vi "Check if configuration files exist.vi"(8 "error in (no error)":errorcluster, 11 "TomoConversionBase in":refnum<class "TomoConversion.lvclass">) -> (0 "error out":errorcluster, 2 "configuration file exists?":bool, 3 "TomoConversionBase out":refnum<class "TomoConversion.lvclass">)   [LabVIEW 2012, in "TomoConversion.lvclass"]
doc: "Checks whether all required configuration files for the component exist."
uses:
  TomoConversion.lvclass
  <vilib>/Distrio/Murmex/Murmex/Murmex.lvclass
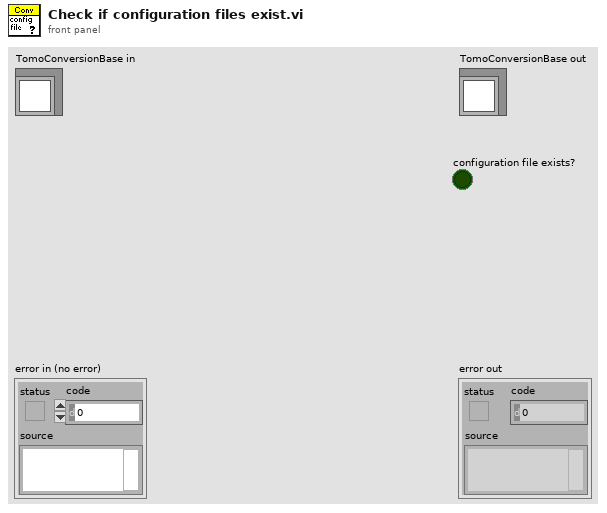
[diagram p1: front panel]
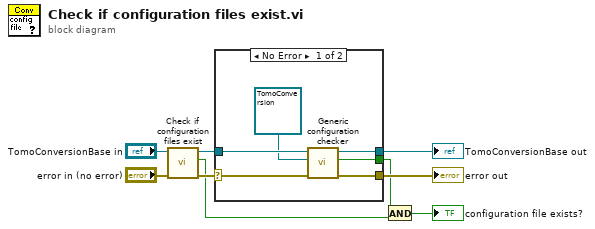
[diagram p0: block diagram]
diagram:
  n1 = call-parent "Check if configuration files exist.vi"("error in (no error)"="error in (no error)", "MurmexBase in"="TomoConversionBase in") -> ("error out"=w7:errorcluster, "configuration file exists?"=w1:bool, "MurmexBase out"=w6:refnum<class "TomoConversion.lvclass">)  [unwired: 7 in]
  n2 = case shown="No Error" w7 {
    selector: w7 -> [w14 w17]
    tunnel: w6 -> [w15 w16]
    tunnel: [w13 w17] -> w5
    tunnel: [w12 w16] -> w4
    tunnel: [w10 _] -> w2
    frame No Error {
      n3 = call <vilib>:"Generic configuration checker.vi"("error in (no error)"=w14, "inheritance level"=refnum<class "TomoConversion.lvclass"> refnum ("TomoConversionBase in"), "Murmex in"=w15) -> ("error out"=w13:errorcluster, "configuration file exists?"=w10:bool, "Murmex out"=w12:refnum<class "TomoConversion.lvclass">)  [unwired: 6 in]
    }
    frame Error {
    }
  }
  "error out" <- w5
  "TomoConversionBase out" <- w4
  n4 = And(x=w2, y=w1) -> (x .and. y?=→"configuration file exists?":bool)
